vi "Handle Value Change.vi"(5 "VolatusAPI":refnum<class "VolatusAPI.lvclass">, 7 "CtlRef":refnum<vi>, 8 "error in (no error)":errorcluster, 9 "NewVal":variant, 10 "OldVal":variant, 11 "HistorianCharting in":refnum<class "HistorianCharting.lvclass">) -> (0 "error out":errorcluster, 3 "HistorianCharting out":refnum<class "HistorianCharting.lvclass">)   [LabVIEW 2020, in "VolatusGUIElements.lvlib" / "HistorianCharting.lvclass"]
uses:
  HistorianCharting.lvclass
  Volatus/VolatusAPI/VolatusAPI.lvclass
  HistorianCharting.lvclass/HistorianCharting.ctl
  Time Data.ctl
  Lock Now Data.ctl
  Config Data.ctl
  Plot Visible Data.ctl
  VolatusGUI/Historian Charting Manager/Scale.ctl
  Scale Data.ctl
  Plot Color Data.ctl
  Selection Data.ctl
  VolatusGUI/Historian Charting Manager/Historian Charting Manager.lvclass
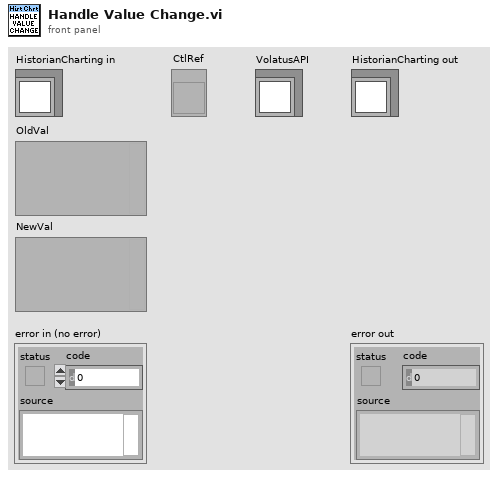
[diagram p1: front panel]
types:
  T1 = cluster{"Config":bool, "Time":string, "Lock Time":bool, "Plots":cluster{"Channel":string, "Value":dbl, "Color":u32, "Scale":bool, "Visible":bool}[], "Graph":cluster{dbl[], dbl[]}[], "Selection":string}
  T2 = typedef "VolatusGUIElements.lvlib/HistorianCharting.lvclass/Time Data.ctl" = cluster{"New Time":string, "Old Time":string}
  T3 = typedef "VolatusGUIElements.lvlib/HistorianCharting.lvclass/Lock Now Data.ctl" = cluster{"Lock Now":bool}
  T4 = typedef "VolatusGUIElements.lvlib/HistorianCharting.lvclass/Config Data.ctl" = cluster{"Unused":bool}
  T5 = cluster{"Channel":string, "Value":dbl, "Color":u32, "Scale":bool, "Visible":bool}[]
  T6 = typedef "VolatusGUIElements.lvlib/HistorianCharting.lvclass/Plot Visible Data.ctl" = cluster{"Index":i32, "Visible":bool}
  T7 = typedef "VolatusGUIElements.lvlib/HistorianCharting.lvclass/Scale Data.ctl" = cluster{"Index":i32, "Scale":T8}
  T8 = typedef "VolatusGUI.lvlib/Historian Charting Manager.lvclass/Scale.ctl" = enum16{"Left", "Right"}
  T9 = typedef "VolatusGUIElements.lvlib/HistorianCharting.lvclass/Plot Color Data.ctl" = cluster{"Index":i32, "Color":u32}
  T10 = typedef "VolatusGUIElements.lvlib/HistorianCharting.lvclass/Selection Data.ctl" = cluster{"Plot Group":string}
  T11 = cluster{"Channel":bool, "Value":bool, "Color":bool, "Scale":bool, "Visible":bool}[]
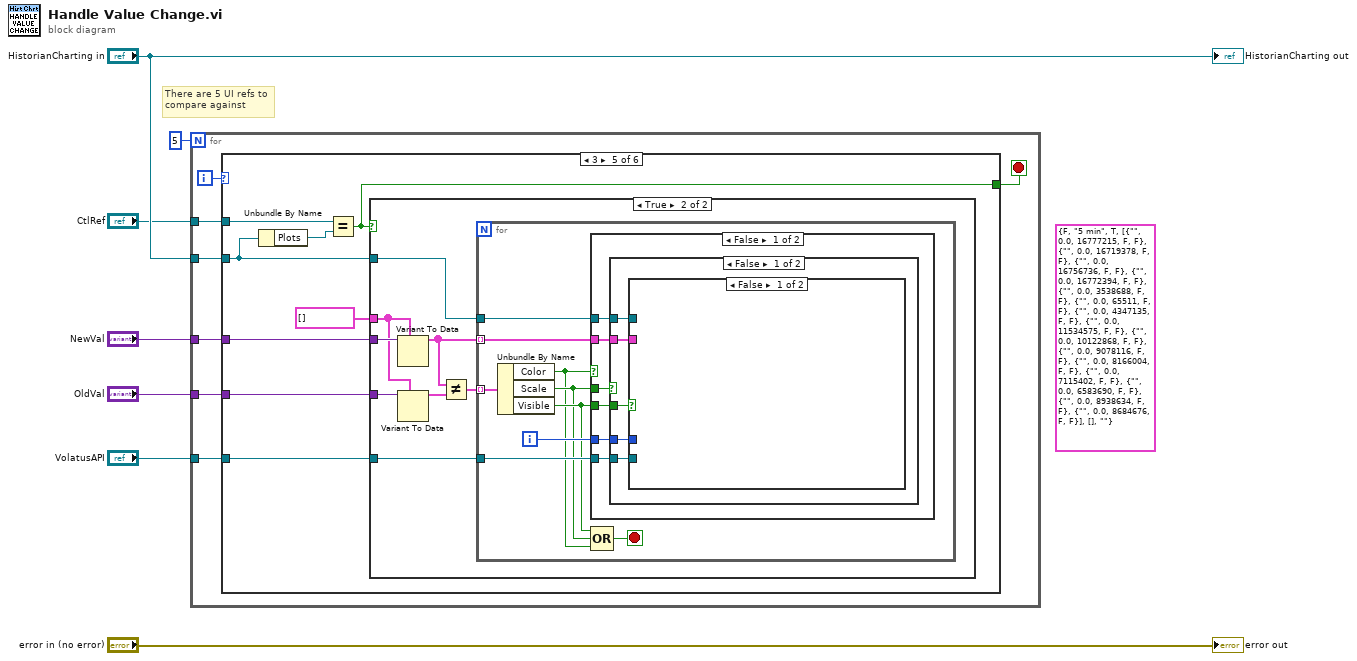
[diagram p0: block diagram]
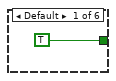
[diagram p2: hidden frame]
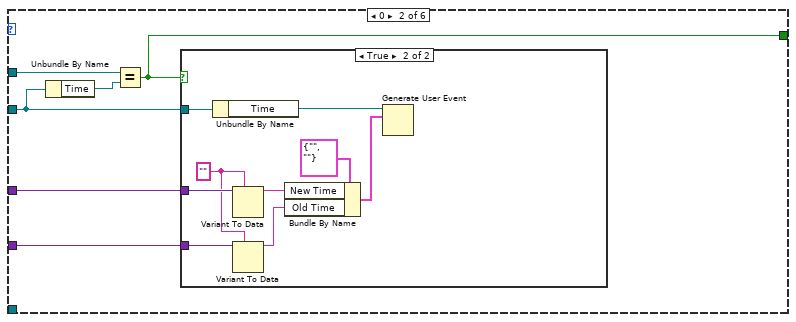
[diagram p3: hidden frame]
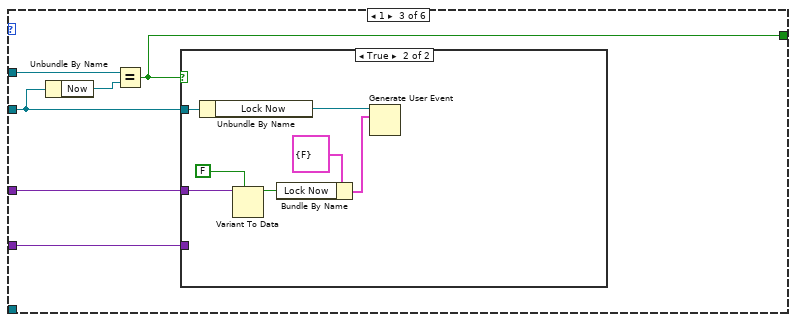
[diagram p5: hidden frame]
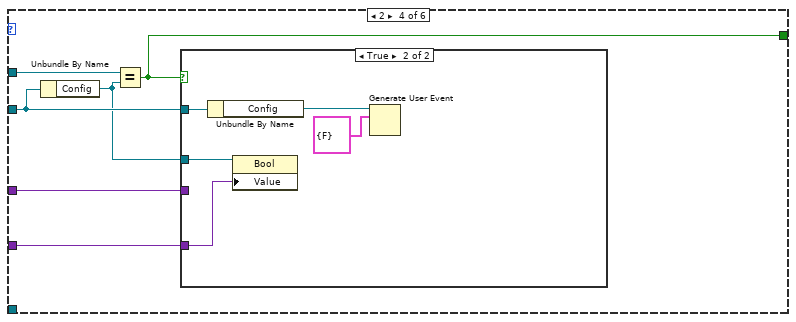
[diagram p7: hidden frame]
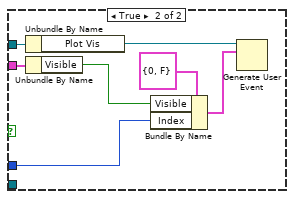
[diagram p10: hidden frame]
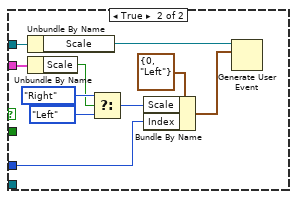
[diagram p11: hidden frame]
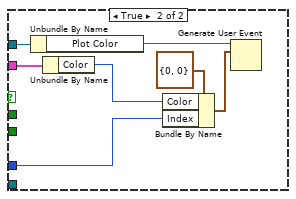
[diagram p12: hidden frame]
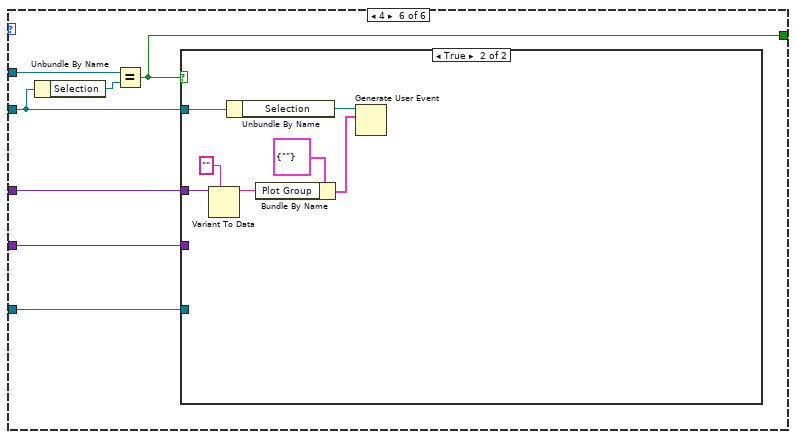
[diagram p13: hidden frame]
diagram:
  (unwired) T1 {"Config"=FALSE, "Time"="5 min", "Lock Time"=TRUE, "Plots"=[{"Channel"="", "Value"=0.0, "Color"=16777215, "Scale"=FALSE, "Visible"=FALSE}, {"Channel"="", "Value"=0.0, "Color"=16719378, "Scale"=FALSE, "Visible"=FALSE}, {"Channel"="", "Value"=0.0, "Color"=16756736, "Scale"=FALSE, "Visible"=FALSE}, {"Channel"="", "Value"=0.0, "Color"=16772394, "Scale"=FALSE, "Visible"=FALSE}, {"Channel"="", "Value"=0.0, "Color"=3538688, "Scale"=FALSE, "Visible"=FALSE}, {"Channel"="", "Value"=0.0, "Color"=65511, "Scale"=FALSE, "Visible"=FALSE}, {"Channel"="", "Value"=0.0, "Color"=4347135, "Scale"=FALSE, "Visible"=FALSE}, {"Channel"="", "Value"=0.0, "Color"=11534575, "Scale"=FALSE, "Visible"=FALSE}, {"Channel"="", "Value"=0.0, "Color"=10122868, "Scale"=FALSE, "Visible"=FALSE}, {"Channel"="", "Value"=0.0, "Color"=9078116, "Scale"=FALSE, "Visible"=FALSE}, {"Channel"="", "Value"=0.0, "Color"=8166004, "Scale"=FALSE, "Visible"=FALSE}, {"Channel"="", "Value"=0.0, "Color"=7115402, "Scale"=FALSE, "Visible"=FALSE}, {"Channel"="", "Value"=0.0, "Color"=6583690, "Scale"=FALSE, "Visible"=FALSE}, {"Channel"="", "Value"=0.0, "Color"=8938634, "Scale"=FALSE, "Visible"=FALSE}, {"Channel"="", "Value"=0.0, "Color"=8684676, "Scale"=FALSE, "Visible"=FALSE}], "Graph"=[], "Selection"=""} ("HistorianChart")
  # "There are 5 UI refs to compare against"
  n1 = for {
    N: 5 -> [_]
    tunnel: "HistorianCharting in" -> [w13]
    tunnel: "NewVal" -> [w9]
    tunnel: "OldVal" -> [w10]
    tunnel: "CtlRef" -> [w12]
    tunnel: "VolatusAPI" -> [w8]
    i -> [w14]
    stop <- w11 stop-if-true
    n2 = case shown="3" w14 {
      tunnel: w13 -> [_ w16 w31 w45 w57 w116]
      tunnel: w12 -> [_ w21 w36 w49 w62 w121]
      tunnel: [TRUE w19 w34 w48 w60 w119] -> w11
      tunnel: w10 -> [_ w18 w33 w47 w59 w118]
      tunnel: w9 -> [_ w17 w32 w46 w58 w117]
      tunnel: w8 -> [_ _ _ _ w55 w115]
      frame Default {
      }
      frame 0 {
        n3 = Unbundle By Name(w16) -> ("Time"=w20:refnum<vi>)
        n4 = Equal?(x=w21, y=w20) -> (x = y?=w19:bool)
        n5 = case shown="True" w19 {
          tunnel: w18 -> [_ w29]
          tunnel: w17 -> [_ w30]
          tunnel: w16 -> [_ w27]
          frame False {
          }
          frame True {
            w28 = ""
            n6 = Unbundle By Name(w27) -> ("Time"=w26:refnum<user-event>)
            n7 = Variant To Data(type=w28, Variant=w30) -> (data=w23:string)  [unwired: 1 in, 1 out]
            n8 = Variant To Data(type=w28, Variant=w29) -> (data=w22:string)  [unwired: 1 in, 1 out]
            n9 = Bundle By Name(cluster=T2 {"New Time"="", "Old Time"=""} ("event data"), "New Time"=w23, "Old Time"=w22) -> (w24:T2)
            n10 = Generate User Event(user event=w26, event data cluster=w24) -> ()  [unwired: 2 in, 2 out]
          }
        }
      }
      frame 1 {
        n11 = Unbundle By Name(w31) -> ("Now"=w35:refnum<vi>)
        n12 = Equal?(x=w36, y=w35) -> (x = y?=w34:bool)
        n13 = case shown="True" w34 {
          tunnel: w33 -> [_ _]
          tunnel: w32 -> [_ w43]
          tunnel: w31 -> [_ w41]
          frame False {
          }
          frame True {
            n14 = Unbundle By Name(w41) -> ("Lock Now"=w40:refnum<user-event>)
            n15 = Variant To Data(type=FALSE, Variant=w43) -> (data=w37:bool)  [unwired: 1 in, 1 out]
            n16 = Bundle By Name(cluster=T3 {"Lock Now"=FALSE} ("event data"), "Lock Now"=w37) -> (w38:T3)
            n17 = Generate User Event(user event=w40, event data cluster=w38) -> ()  [unwired: 2 in, 2 out]
          }
        }
      }
      frame 2 {
        n18 = Unbundle By Name(w45) -> ("Config"=w44:refnum<vi>)
        n19 = Equal?(x=w49, y=w44) -> (x = y?=w48:bool)
        n20 = case shown="True" w48 {
          tunnel: w47 -> [_ w51]
          tunnel: w46 -> [_ _]
          tunnel: w45 -> [_ w54]
          tunnel: w44 -> [_ w52]
          frame False {
          }
          frame True {
            n21 = Unbundle By Name(w54) -> ("Config"=w53:refnum<user-event>)
            n22 = property class="Bool"(reference=w52, "Value"=w51) -> ()  [unwired: 1 in, 2 out]
            n23 = Generate User Event(user event=w53, event data cluster=T4 {"Unused"=FALSE} ("event data")) -> ()  [unwired: 2 in, 2 out]
          }
        }
      }
      frame 3 {
        n24 = Unbundle By Name(w57) -> ("Plots"=w61:refnum<vi>)
        n25 = Equal?(x=w62, y=w61) -> (x = y?=w60:bool)
        n26 = case shown="True" w60 {
          tunnel: w59 -> [_ w69]
          tunnel: w58 -> [_ w70]
          tunnel: w57 -> [_ w64]
          tunnel: T5 [] ("Plots") -> [_ w68]
          tunnel: w55 -> [_ w63]
          frame False {
          }
          frame True {
            n27 = Variant To Data(type=w68, Variant=w70) -> (data=w65:T5)  [unwired: 1 in, 1 out]
            n28 = Variant To Data(type=w68, Variant=w69) -> (data=w67:T5)  [unwired: 1 in, 1 out]
            n29 = Not Equal?(x=w65, y=w67) -> (x != y?=w66:T11)
            n30 = for {
              tunnel: w66 -> [w79] mode=indexing
              tunnel: w65 -> [w78] mode=indexing
              tunnel: w64 -> [w77]
              tunnel: w63 -> [w75]
              i -> [w76]
              stop <- w71 stop-if-true
              n31 = Unbundle By Name(w79) -> ("Color"=w72:bool, "Scale"=w73:bool, "Visible"=w74:bool)
              n32 = case shown="False" w72 {
                tunnel: w73 -> [w85 _]
                tunnel: w74 -> [w84 _]
                tunnel: w78 -> [w82 w114]
                tunnel: w77 -> [w81 w113]
                tunnel: w76 -> [w83 w108]
                tunnel: w75 -> [w80 _]
                frame False {
                  n33 = case shown="False" w85 {
                    tunnel: w84 -> [w90 _]
                    tunnel: w83 -> [w89 w98]
                    tunnel: w82 -> [w88 w107]
                    tunnel: w81 -> [w87 w103]
                    tunnel: w80 -> [w86 _]
                    frame False {
                      n34 = case shown="False" w90 {
                        tunnel: w89 -> [_ w91]
                        tunnel: w88 -> [_ w97]
                        tunnel: w87 -> [_ w96]
                        tunnel: w86 -> [_ _]
                        frame False {
                        }
                        frame True {
                          n35 = Unbundle By Name(w96) -> ("Plot Vis"=w95:refnum<user-event>)
                          n36 = Unbundle By Name(w97) -> ("Visible"=w92:bool)
                          n37 = Bundle By Name(cluster=T6 {"Index"=0, "Visible"=FALSE} ("event data"), "Visible"=w92, "Index"=w91) -> (w93:T6)
                          n38 = Generate User Event(user event=w95, event data cluster=w93) -> ()  [unwired: 2 in, 2 out]
                        }
                      }
                    }
                    frame True {
                      n39 = Unbundle By Name(w103) -> ("Scale"=w102:refnum<user-event>)
                      n40 = Unbundle By Name(w107) -> ("Scale"=w104:bool)
                      n41 = Select(t=Scale."Right" ("Scale"), s=w104, f=Scale."Left" ("Scale")) -> (s? t:f=w99:T8)
                      n42 = Bundle By Name(cluster=T7 {"Index"=0, "Scale"=enum."Left"} ("event data"), "Scale"=w99, "Index"=w98) -> (w100:T7)
                      n43 = Generate User Event(user event=w102, event data cluster=w100) -> ()  [unwired: 2 in, 2 out]
                    }
                  }
                }
                frame True {
                  n44 = Unbundle By Name(w113) -> ("Plot Color"=w112:refnum<user-event>)
                  n45 = Unbundle By Name(w114) -> ("Color"=w109:u32)
                  n46 = Bundle By Name(cluster=T9 {"Index"=0, "Color"=0} ("event data"), "Color"=w109, "Index"=w108) -> (w110:T9)
                  n47 = Generate User Event(user event=w112, event data cluster=w110) -> ()  [unwired: 2 in, 2 out]
                }
              }
              n48 = Compound Arithmetic op=OR(w74, w73, w72) -> (w71:bool)
            }
          }
        }
      }
      frame 4 {
        n49 = Unbundle By Name(w116) -> ("Selection"=w120:refnum<vi>)
        n50 = Equal?(x=w121, y=w120) -> (x = y?=w119:bool)
        n51 = case shown="True" w119 {
          tunnel: w118 -> [_ _]
          tunnel: w117 -> [_ w128]
          tunnel: w116 -> [_ w126]
          tunnel: w115 -> [_ _]
          frame False {
          }
          frame True {
            n52 = Variant To Data(type="", Variant=w128) -> (data=w122:string)  [unwired: 1 in, 1 out]
            n53 = Unbundle By Name(w126) -> ("Selection"=w125:refnum<user-event>)
            n54 = Bundle By Name(cluster=T10 {"Plot Group"=""} ("event data"), "Plot Group"=w122) -> (w123:T10)
            n55 = Generate User Event(user event=w125, event data cluster=w123) -> ()  [unwired: 2 in, 2 out]
          }
        }
      }
    }
  }
  "error out" <- "error in (no error)"
  "HistorianCharting out" <- "HistorianCharting in"
